vi "Add Data Record.vi"(3 "Data In":dbl[][](array[numeric]) format="%.2f", 4 "Data to update":dbl[](array[numeric]) format="%.2f", 5 "Index":i32) -> (0 "Data Display":string, 2 "Data Out":dbl[][](array[numeric]) format="%.2f")   [LabVIEW 2021]
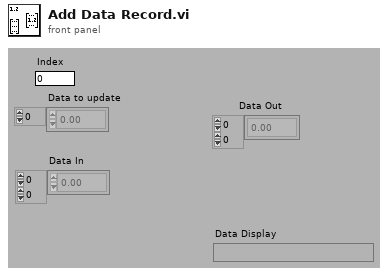
[diagram p1: front panel]
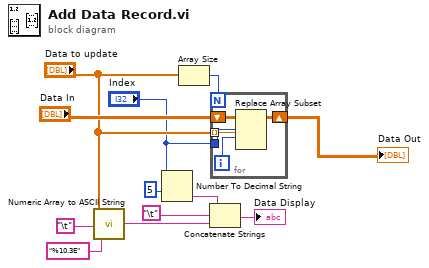
[diagram p0: block diagram]
diagram:
  n1 = call "Numeric Array to ASCII String.vi"("format string"="%10.3E", "delimiter"="\t", "numeric array"="Data to update") -> ("ascii string"=w10:string)
  n2 = Number To Decimal String(number="Index", width (-)=5) -> (decimal integer string=w6:string)
  n3 = Array Size(array="Data to update") -> (size(s)=w9:i32)
  n4 = Concatenate Strings(w6, "\t", w10) -> (→"Data Display":string)
  n5 = for {
    N: w9 -> [_]
    shift-right: [w17] -> w4
    shift-left: "Data In" -> [w13]
    tunnel: "Index" -> [w14]
    tunnel: "Data to update" -> [w16] mode=indexing
    i -> [w15]
    n6 = Replace Array Subset(array=w13, new element=w16, index (row)=w14, index (col)=w15) -> (w17:dbl[][])
  }
  "Data Out" <- w4
